vi "电导率_所有参数读取.vi"(8 "error in (no error)":errorcluster caption="错误输入（无错误）", 11 "MB session in":refnum<class "MB_Master.lvclass">) -> (0 "error out":errorcluster caption="错误输出", 2 "输出值":T1 {"电极型号标志" items=["NULL", "pH", "Cond", "DO", "Turb"]; "电极状态标志" items=["OK"]}, 3 "MB session out":refnum<class "MB_Master.lvclass">)   [LabVIEW 2016, in "斯坦道多参数.lvlib"]
uses:
  <vilib>/Plasmionique/MB Master/MB_Master/MB_Master.lvclass
  <vilib>/Plasmionique/MB Master/MB Master.lvlib
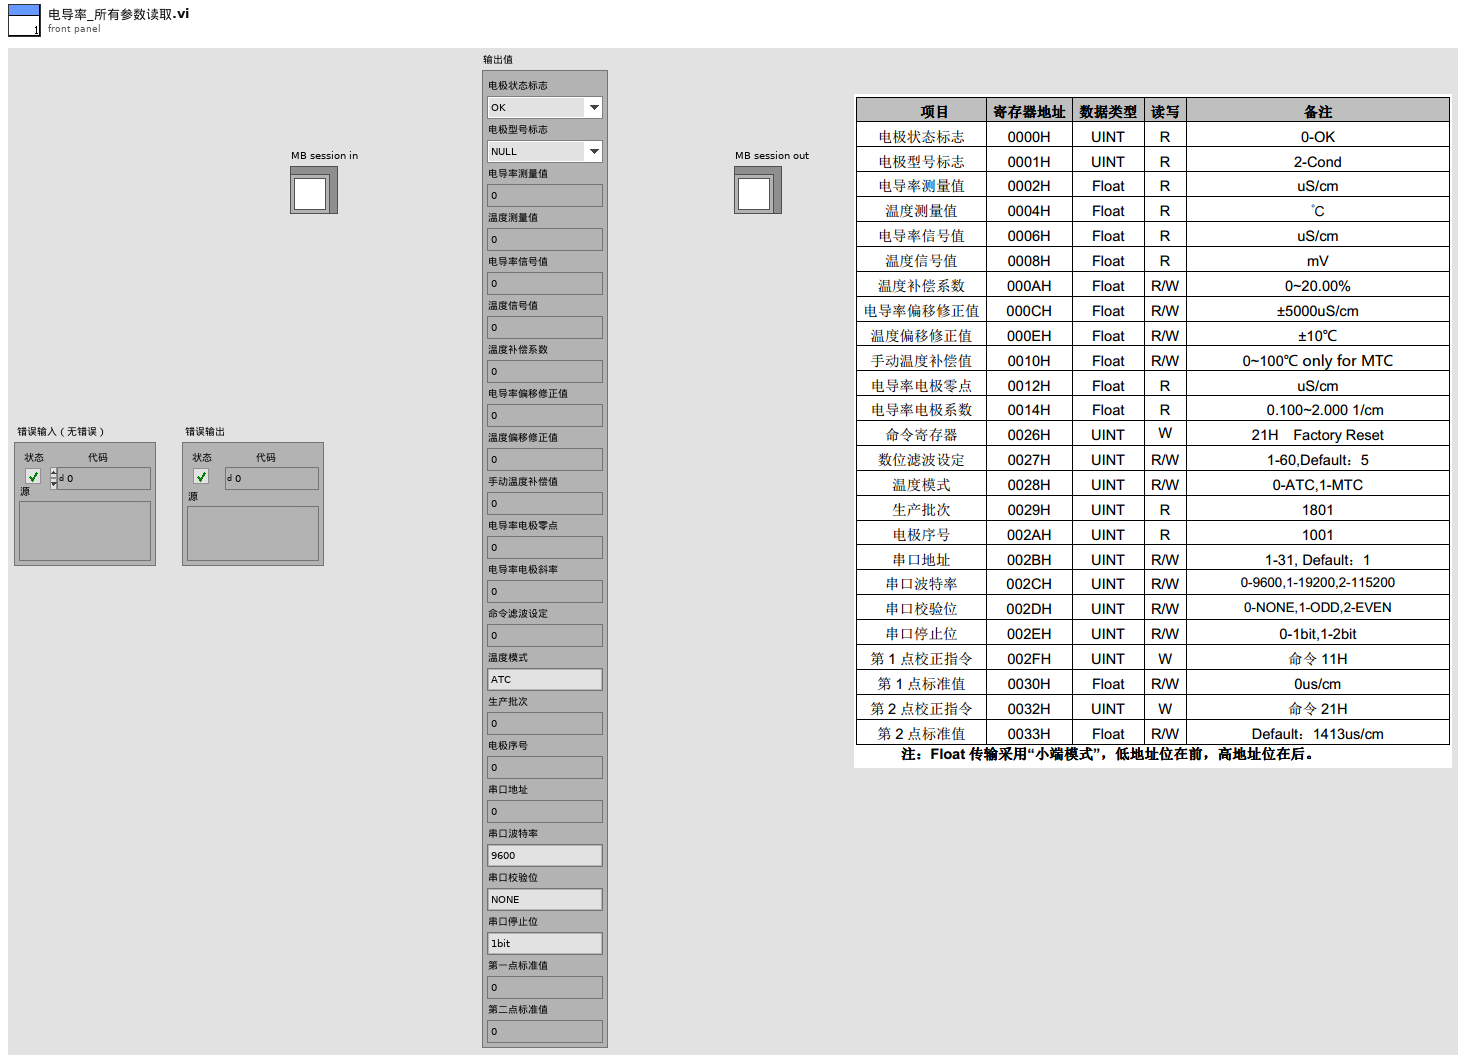
[diagram p1: front panel]
types:
  T1 = cluster{"电极状态标志":u16, "电极型号标志":u16, "电导率测量值":sgl, "温度测量值":sgl, "电导率信号值":sgl, "温度信号值":sgl, "温度补偿系数":sgl, "电导率偏移修正值":sgl, "温度偏移修正值":sgl, "手动温度补偿值":sgl, "电导率电极零点":sgl, "电导率电极斜率":sgl, "命令滤波设定":u16, "温度模式":enum16{"ATC", "MTC"}, "生产批次":u16, "电极序号":u16, "串口地址":u16, "串口波特率":enum16{"9600", "19200", "115200"}, "串口校验位":enum16{"NONE", "ODD", "EVEN"}, "串口停止位":enum16{"1bit", "2bit"}, "第一点标准值":sgl, "第二点标准值":sgl}
  T2 = cluster{u16, u16, "数值":sgl, "数值":sgl, "数值":sgl, "数值":sgl, "数值":sgl, "数值":sgl, "数值":sgl, "数值":sgl, "数值":sgl, "数值":sgl, u16, u16, u16, u16, u16, u16, u16, u16, "数值":sgl, "数值":sgl}
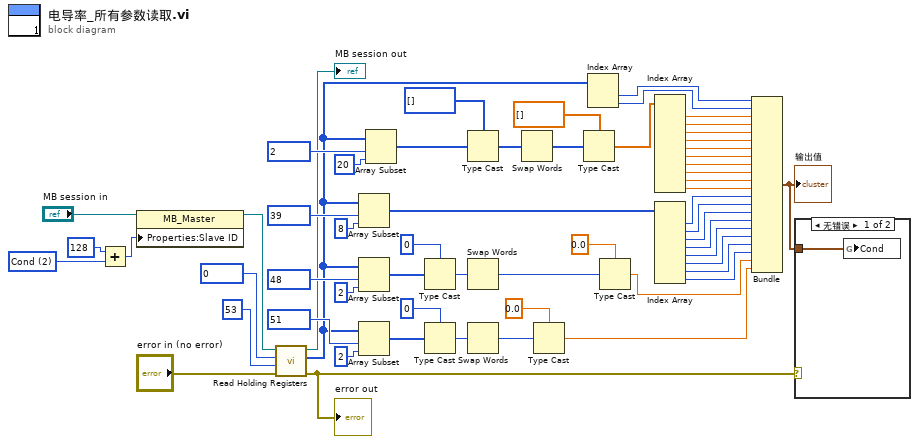
[diagram p0: block diagram]
diagram:
  w59 = u16 2 items=["NULL", "pH", "Cond", "DO", "Turb"] ("数值")
  n1 = Add(x=u16 128, y=w59) -> (x+y=w58:u16)
  n2 = property class="MB_Master"(reference="MB session in", "Properties:Slave ID"=w58) -> (reference out=w11:refnum<class "MB_Master.lvclass">)  [unwired: 1 in, 1 out]
  n3 = call <vilib>:"Read Holding Registers.vi"("error in (no error)"="error in (no error)", "quantity"=u16 53, "starting address"=u16 0, "MB session in"=w11) -> ("error out"=w4:errorcluster, "Registers"=w25:u16[], "MB session out"=→"MB session out":refnum<class "MB_Master.lvclass">)  [unwired: 5 in]
  "error out" <- w4
  n4 = Array Subset(array=w25, index=u16 39 ("starting address"), length=8 ("长度")) -> (w38:u16[])
  n5 = Array Subset(array=w25, index=u16 48 ("starting address"), length=2 ("长度")) -> (w20:u16[])
  n6 = Array Subset(array=w25, index=u16 51 ("starting address"), length=2 ("长度")) -> (w15:u16[])
  n7 = Array Subset(array=w25, index=u16 2 ("starting address"), length=20 ("长度")) -> (w47:u16[])
  n8 = Type Cast(type=u32 0 ("数值"), x=w20) -> (*(type *) &x=w23:u32)
  n9 = Type Cast(type=u32 0 ("数值"), x=w15) -> (*(type *) &x=w17:u32)
  n10 = Type Cast(type=u32[] [] ("数组 2"), x=w47) -> (*(type *) &x=w49:u32[])
  n11 = Swap Words(1:w23) -> (0:w24:u32)
  n12 = Swap Words(1:w17) -> (0:w16:u32)
  n13 = Swap Words(1:w49) -> (0:w51:u32[])
  n14 = Type Cast(type=sgl 0.0 ("数值"), x=w16) -> (*(type *) &x=w13:sgl)
  n15 = Type Cast(type=sgl[] [] ("数组 2"), x=w51) -> (*(type *) &x=w46:sgl[])
  n16 = Index Array(array=w25) -> (element #1=w54:u16, element #2=w53:u16)  [unwired: 2 in]
  n17 = Type Cast(type=sgl 0.0 ("数值"), x=w24) -> (*(type *) &x=w14:sgl)
  n18 = Index Array(array=w46) -> (element #1=w45:sgl, element #2=w44:sgl, element #3=w43:sgl, element #4=w42:sgl, element #5=w10:sgl, element #6=w9:sgl, element #7=w8:sgl, element #8=w7:sgl, element #9=w6:sgl, element #10=w5:sgl)  [unwired: 10 in]
  n19 = Index Array(array=w38) -> (element #1=w37:u16, element #2=w36:u16, element #3=w35:u16, element #4=w34:u16, element #5=w33:u16, element #6=w32:u16, element #7=w31:u16, element #8=w30:u16)  [unwired: 8 in]
  n20 = Bundle(w54, w53, "数值"=w45, "数值"=w44, "数值"=w43, "数值"=w42, "数值"=w10, "数值"=w9, "数值"=w8, "数值"=w7, "数值"=w6, "数值"=w5, w37, w36, w35, w34, w33, w32, w31, w30, "数值"=w14, "数值"=w13) -> (w3:T2)  [unwired: 1 in]
  "输出值" <- w3
  n21 = case shown="无错误" w4 {
    tunnel: w3 -> [w60 _]
    frame No Error {
      n22 = global write "国弘过程全局变量.vi" "Cond"(w60) -> ()
    }
    frame Error {
    }
  }
